vi "Main.vi"(8 "error in (no error)":errorcluster, 11 "VISA resource name":refnum<visa-resource-name>) -> (0 "error out":errorcluster, 2 "read buffer":string)   [LabVIEW 2016]
uses:
  <vilib>/Instr/_visa.llb/VISA Configure Serial Port (Instr).vi
panel:
  in  "stop":bool
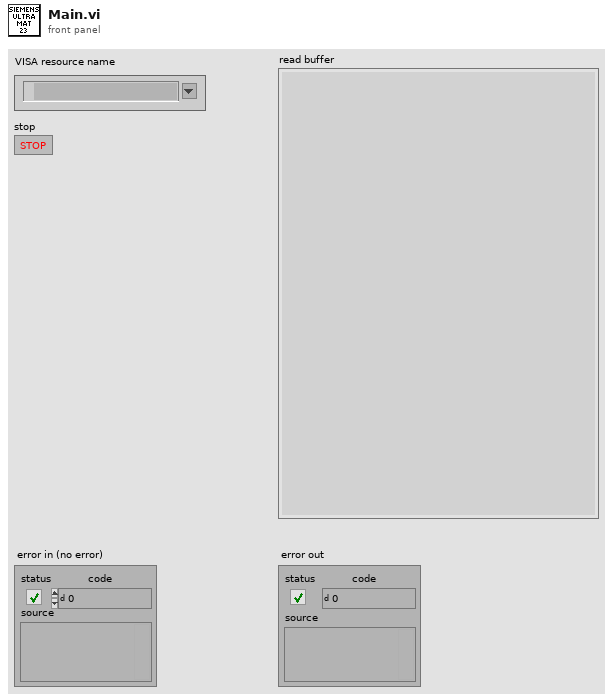
[diagram p1: front panel]
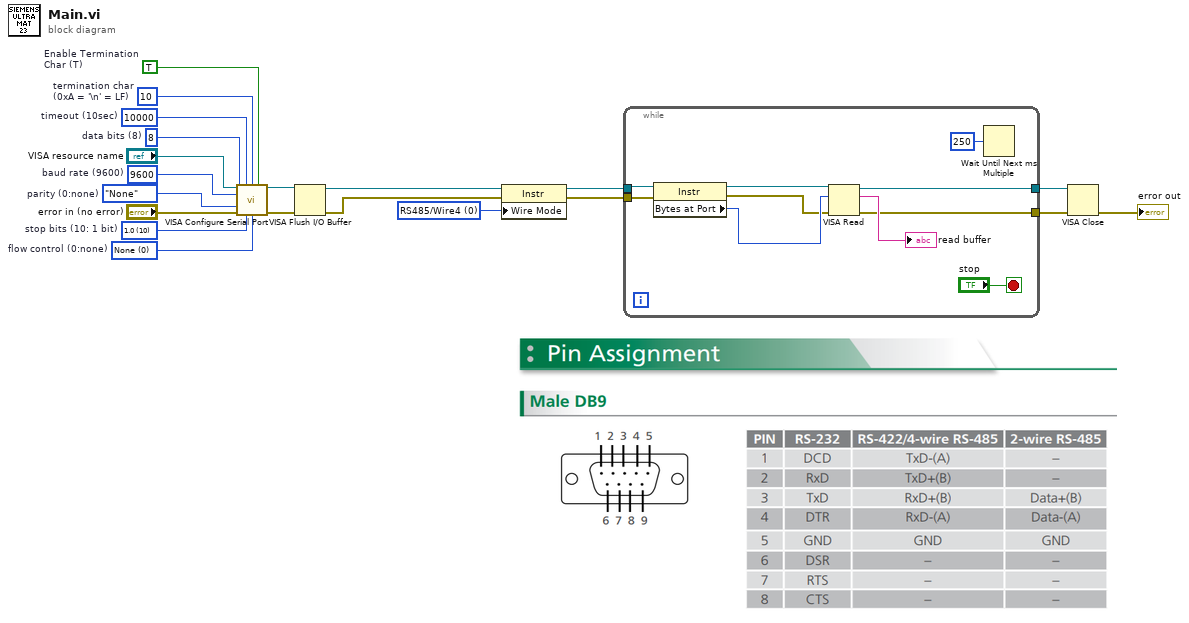
[diagram p0: block diagram]
diagram:
  w4 = TRUE  # Enable Termination Char (T)
  w5 = u8 10  # termination char (0xA = '\n' = LF)
  w6 = u32 10000  # timeout (10sec)
  w7 = u16 0 items=["None", "XON/XOFF", "RTS/CTS", "XON/XOFF & RTS/CTS", "DTR/DSR", "XON/XOFF & DTR/DSR"]  # flow control (0:none)
  w8 = u16 10 items=["1.0"=10, "1.5"=15, "2.0"=20]  # stop bits (10: 1 bit)
  w9 = enum16{"None", "Odd", "Even", "Mark", "Space"}."None"  # parity (0:none)
  w10 = u16 8  # data bits (8)
  w11 = u32 9600  # baud rate (9600)
  w20 = i16 0 items=["Unknown"=-1, "RS485/Wire4"=0, "RS485/Wire2-EchoDTR"=1, "RS485/Wire2-CtrlDTR"=2, "RS485/Wire2-Auto"=3, "RS232/DTE"=128, "RS232/DCE"=129, "RS232/Auto"=130] ("Serial Settings:Wire Mode")
  n1 = call-poly "VISA Configure Serial Port"("VISA resource name"="VISA resource name", "timeout (10sec)"=w6, "termination char\n(0xA = '\\n' = LF)"=w5, "Enable Termination\nChar (T)"=w4, "baud rate (9600)"=w11, "data bits (8)"=w10, "parity (0:none)"=w9, "error in (no error)"="error in (no error)", "stop bits (10: 1 bit)"=w8, "flow control (0:none)"=w7) -> ("VISA resource name out"=w15:refnum<visa-resource-name>, "error out"=w17:errorcluster)  [unwired: 4 in]
  n2 = VISA Flush I/O Buffer(VISA resource name=w15, error in (no error)=w17) -> (VISA resource name out=w14:refnum<visa-resource-name>, error out=w16:errorcluster)  [unwired: 1 in]
  n3 = property class="Instr"(reference=w14, error in=w16, "Wire Mode"=w20) -> (reference out=w19:refnum<visa-resource-name>, error out=w18:errorcluster)
  n4 = while {
    tunnel: w19 -> [w30]
    tunnel: w18 -> [w29]
    tunnel: [w26] -> w12
    tunnel: [w22] -> w13
    stop <- "stop" stop-if-true
    n5 = property class="Instr"(reference=w30, error in=w29) -> (reference out=w28:refnum<visa-resource-name>, error out=w21:errorcluster, "Bytes at Port"=w27:u32)
    n6 = VISA Read(VISA resource name=w28, byte count=w27, error in (no error)=w21) -> (VISA resource name out=w26:refnum<visa-resource-name>, read buffer=→"read buffer":string, error out=w22:errorcluster)  [unwired: 1 out]
    n7 = Wait Until Next ms Multiple(millisecond multiple=u32 250) -> ()  [unwired: 1 out]
  }
  n8 = VISA Close(VISA resource name=w12, error in (no error)=w13) -> (error out=→"error out":errorcluster)
